vi "Backward with Scale.vi"(9 "Scale factor":dbl[](array[numeric]), 10 "O Observed Sequence":i32[](array[numeric]), 11 "HMM Cluster":T1) -> (2 "Beta Partial Probalility":dbl[][](array[numeric]))   [LabVIEW 2014, in "HMM.lvlib"]
doc: "Normalize the partial probability for the backward algorithm."
uses:
  HMM.lvlib
  Control/HMM Cluster.ctl
panel:
  out "Array":dbl[](array[numeric])
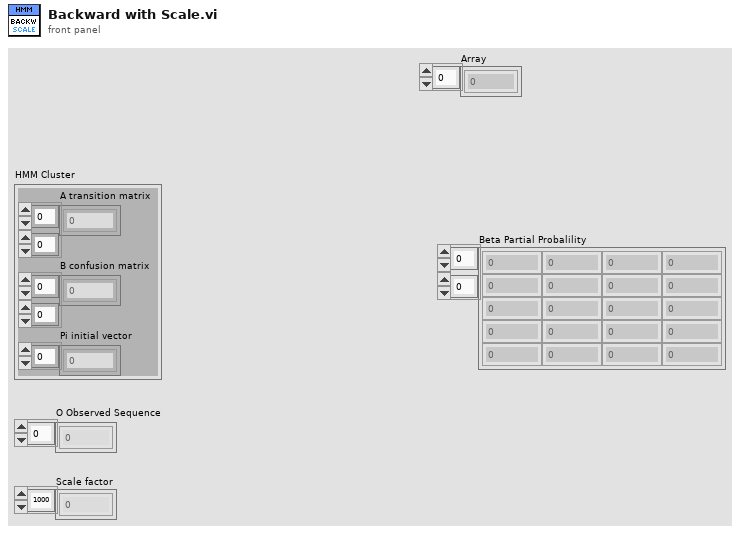
[diagram p1: front panel]
types:
  T1 = typedef "HMM.lvlib/HMM Cluster.ctl" = cluster{"A transition matrix":dbl[][], "B confusion matrix":dbl[][], "Pi initial vector":dbl[]}
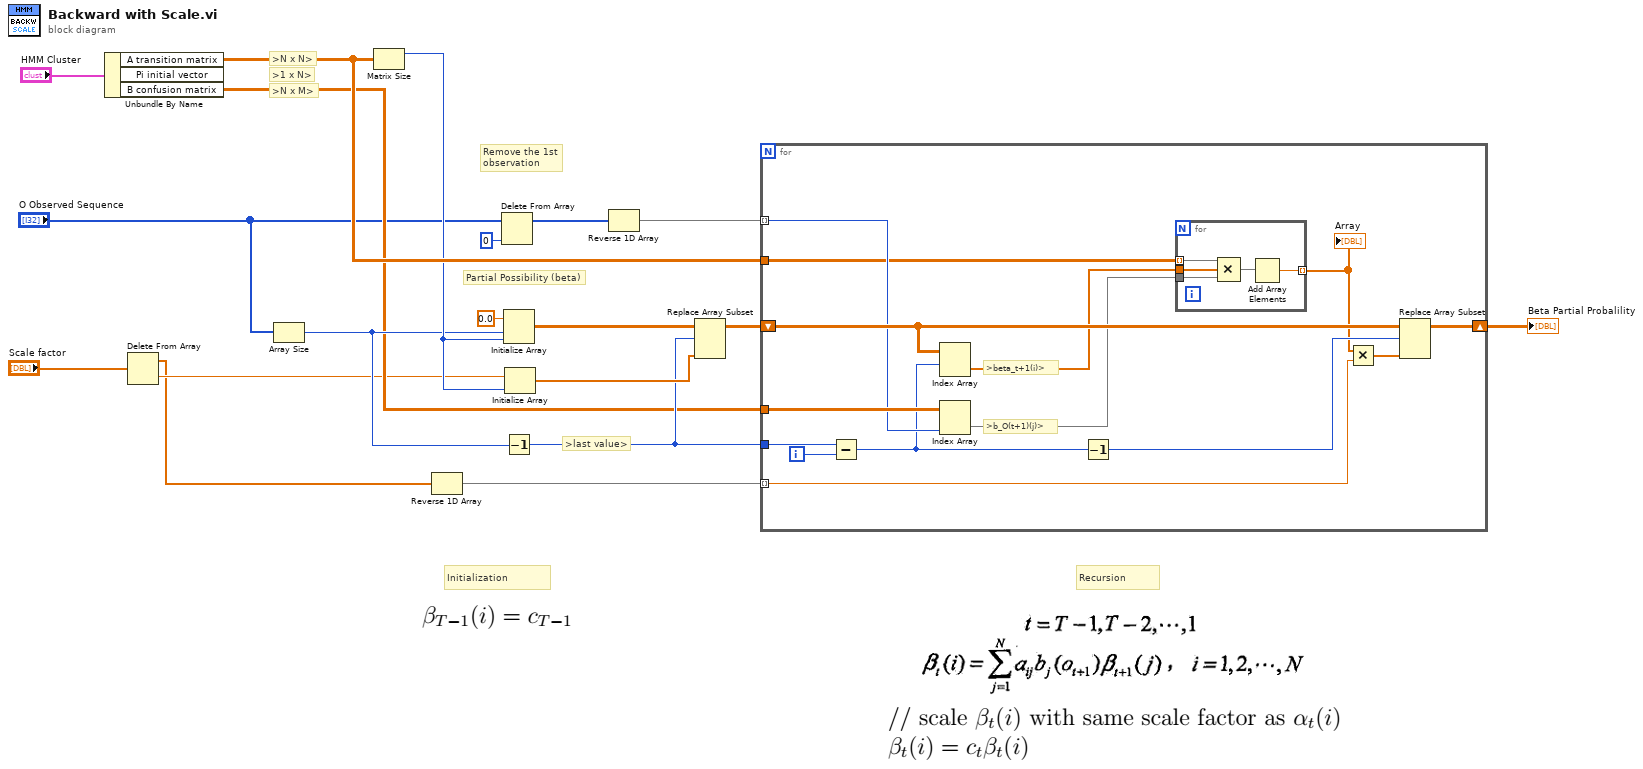
[diagram p0: block diagram]
diagram:
  # "Remove the 1st\nobservation"
  # ">last value>"
  # "Recursion"
  # "Initialization"
  # ">N x M>"
  # ">1 x N>"
  # ">N x N>"
  # "Partial Possibility (beta)"
  n1 = Unbundle By Name("HMM Cluster") -> ("A transition matrix"=w15:dbl[][], "B confusion matrix"=w8:dbl[][])  [unwired: 1 out]
  n2 = Delete From Array(array="Scale factor") -> (deleted portion=w3:dbl, array with subset deleted=w2:dbl[])  [unwired: 2 in]
  n3 = Array Size(array="O Observed Sequence") -> (size(s)=w11:i32)
  n4 = Matrix Size(0:w15) -> (1:w13:i32)  [unwired: 1 out]
  n5 = Reverse 1D Array(array=w2) -> (reversed array=w1:dbl[])
  n6 = Delete From Array(array="O Observed Sequence", index=0) -> (array with subset deleted=w6:i32[])  [unwired: 1 in, 1 out]
  n7 = Initialize Array(0.0 ("element"), w11, w13) -> (w17:dbl[][])
  n8 = Decrement(x=w11) -> (x-1=w9:i32)
  n9 = Initialize Array(w3, w13) -> (w12:dbl[])
  n10 = Reverse 1D Array(array=w6) -> (reversed array=w10:i32[])
  n11 = Replace Array Subset(array=w17, new element=w12, index (row)=w9) -> (w16:dbl[][])  [unwired: 1 in]
  n12 = for {
    tunnel: w10 -> [w31] mode=indexing
    shift-right: [w27] -> w14
    shift-left: w16 -> [w33]
    tunnel: w15 -> [w25]
    tunnel: w8 -> [w32]
    tunnel: w9 -> [w30]
    tunnel: w1 -> [w20] mode=indexing
    i -> [w26]
    # ">beta_t+1(i)>"
    # ">b_O(t+1)(j)>"
    n13 = Subtract(x=w30, y=w26) -> (x-y=w29:i32)
    n14 = Index Array(array=w33, index (row)=w29) -> (element=w24:dbl[])  [unwired: 1 in]
    n15 = Index Array(array=w32, index (col)=w31) -> (element=w23:dbl[])  [unwired: 1 in]
    n16 = Decrement(x=w29) -> (x-1=w28:i32)
    n17 = for {
      tunnel: w25 -> [w38] mode=indexing
      tunnel: w24 -> [w37]
      tunnel: w23 -> [w36]
      tunnel: [w34] -> w22 mode=indexing
      n18 = Compound Arithmetic op=MULTIPLY(w38, w37, w36) -> (w35:dbl[])
      n19 = Add Array Elements(numeric array=w35) -> (sum=w34:dbl)
    }
    "Array" <- w22
    n20 = Multiply(x=w22, y=w20) -> (x*y=w21:dbl[])
    n21 = Replace Array Subset(array=w33, new element=w21, index (row)=w28) -> (w27:dbl[][])  [unwired: 1 in]
  }
  "Beta Partial Probalility" <- w14
